vi "PiezoOpenSynchronization.vi"(9 "error in (no error)":errorcluster) -> (6 "error out":errorcluster, 7 "PiezoSynchronization":T1)   [LabVIEW 2009]
uses:
  Controls/PiezoSynchronization.ctl
  Controls/PIEZO.COMMAND.QUEUE.ctl
  Controls/PIEZO.COMMAND.ctl
  Controls/PIEZO.COMMANDBASIC.ctl
  Controls/PIEZO.WAVE.ctl
  Controls/PIEZO.STATE.ctl
  Controls/PIEZO.WAVE.NOTIFIER.ctl
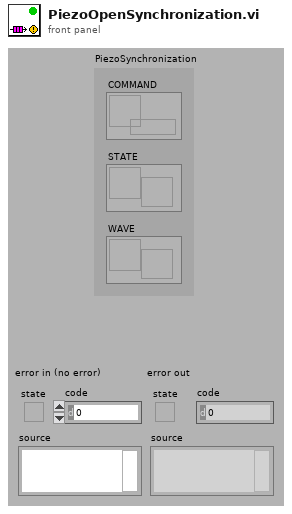
[diagram p1: front panel]
types:
  T1 = typedef "PiezoSynchronization.ctl" = cluster{"COMMAND":T2, "STATE":refnum<notifier>, "WAVE":T3}
  T2 = typedef "PIEZO.COMMAND.QUEUE.ctl" = refnum<queue>
  T3 = typedef "PIEZO.WAVE.NOTIFIER.ctl" = refnum<notifier>
  T4 = typedef "PIEZO.WAVE.ctl" = cluster{"Speed":dbl[unit], "Stiffness (0.95)":dbl, "Linear Stroke":dbl[unit], "Delay":dbl[unit]}
  T5 = typedef "PIEZO.COMMAND.ctl" = cluster{"Command":T6, "WAVE":T4}
  T6 = typedef "PIEZO.COMMANDBASIC.ctl" = enum16{"RUN", "STOP", "QUIT"}
  T7 = typedef "PIEZO.STATE.ctl" = enum16{"IDLE", "STARTING", "RUNNING", "STOPPING", "OFF"}
  T8 = cluster{"queue out":refnum<queue>, "notifier out":refnum<notifier>, "notifier out":refnum<notifier>}
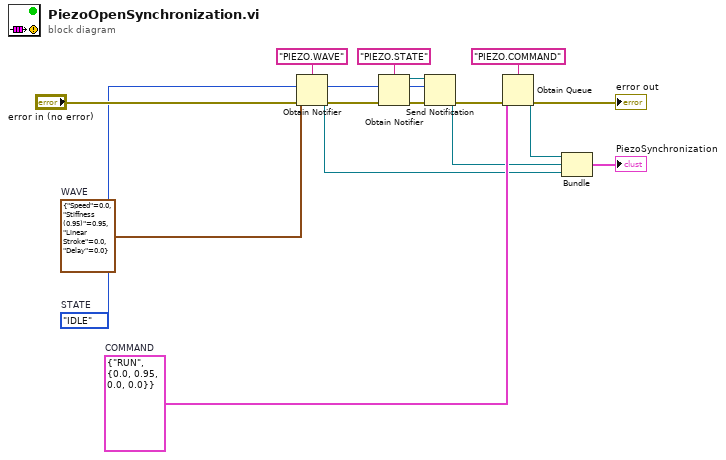
[diagram p0: block diagram]
diagram:
  w7 = T4 {"Speed"=0.0, "Stiffness (0.95)"=0.95, "Linear Stroke"=0.0, "Delay"=0.0}  # WAVE
  w15 = T5 {"Command"=enum."RUN", "WAVE"={"Speed"=0.0, "Stiffness (0.95)"=0.95, "Linear Stroke"=0.0, "Delay"=0.0}}  # COMMAND
  w3 = PIEZO.STATE."IDLE"  # STATE
  n1 = Obtain Notifier(name (unnamed)="PIEZO.WAVE" ("nom (aucun)"), notification data type=w7, error in (no error)="error in (no error)") -> (notifier out=w6:refnum<notifier>, error out=w9:errorcluster)  [unwired: 1 in, 1 out]
  n2 = Obtain Notifier(name (unnamed)="PIEZO.STATE" ("nom (aucun)"), notification data type=w3, error in (no error)=w9) -> (notifier out=w2:refnum<notifier>, error out=w5:errorcluster)  [unwired: 1 in, 1 out]
  n3 = Send Notification(notification=w3, notifier=w2, error in (no error)=w5) -> (notifier out=w1:refnum<notifier>, error out=w4:errorcluster)
  n4 = Obtain Queue(name (unnamed)="PIEZO.COMMAND" ("nom (aucun)"), element data type=w15, error in (no error)=w4) -> (queue out=w13:refnum<queue>, error out=→"error out":errorcluster)  [unwired: 2 in, 1 out]
  n5 = Bundle("queue out"=w13, "notifier out"=w1, "notifier out"=w6) -> (→"PiezoSynchronization":T8)  [unwired: 1 in]
